vi "LabVIEW Versions.vi"() -> (1 "Patch":i32, 2 "Minor":i32, 3 "Major":i32)   [LabVIEW 2020, in "Collector.lvlib" / "LabVIEW Collector.lvclass"]
uses:
  LabVIEW Collector.lvclass
panel:
  out "error out":errorcluster
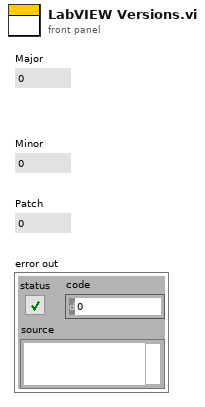
[diagram p1: front panel]
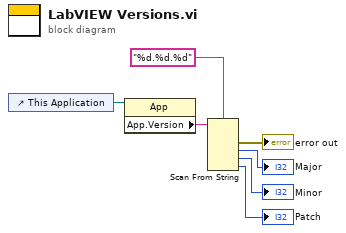
[diagram p0: block diagram]
diagram:
  n1 = control-ref of="This Application"() -> (w1:refnum<vi>)
  n2 = property class="App"(reference=w1) -> ("App.Version"=w3:string)  [unwired: 1 in, 2 out]
  n3 = Scan From String(format string="%d.%d.%d", input string=w3) -> (error out=→"error out":errorcluster, output 1=→"Major":i32, output 2=→"Minor":i32, output 3=→"Patch":i32)  [unwired: 5 in, 2 out]
